vi "等分取数据.vi"(0 "Max":dbl, 1 "MIN":dbl, 3 "num":i32) -> (7 "数据点":dbl[](array[numeric]))   [LabVIEW 2010]
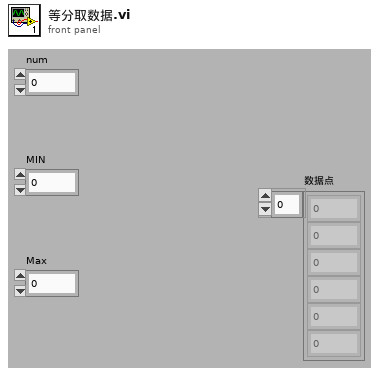
[diagram p1: front panel]
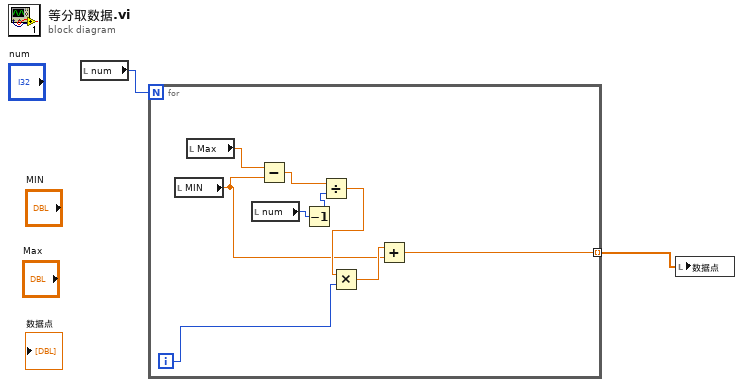
[diagram p0: block diagram]
diagram:
  n1 = local read "num"() -> (w1:i32)
  n2 = for {
    N: w1 -> [_]
    tunnel: [w6] -> w2 mode=indexing
    i -> [w5]
    n3 = local read "MIN"() -> (w7:dbl)
    n4 = local read "Max"() -> (w11:dbl)
    n5 = local read "num"() -> (w4:i32)
    n6 = Subtract(x=w11, y=w7) -> (x-y=w10:dbl)
    n7 = Decrement(x=w4) -> (x-1=w3:i32)
    n8 = Divide(x=w10, y=w3) -> (x/y=w9:dbl)
    n9 = Multiply(x=w9, y=w5) -> (x*y=w8:dbl)
    n10 = Add(x=w8, y=w7) -> (x+y=w6:dbl)
  }
  n11 = local write "数据点"(w2) -> ()
